vi "Read Col Data.vi"(7 "Section Name":string, 8 "error in (no error)":errorcluster, 10 "Col Header Name":string, 11 "Config Data":T1(array[cluster])) -> (0 "error out":errorcluster, 1 "Column Data":string[](array[string]), 3 "Config Data dup":T1(array[cluster]), 4 "Key Find?":bool)   [LabVIEW 2020, in "GUCalibration2.lvlib"]
uses:
  GUCalibration2.lvlib
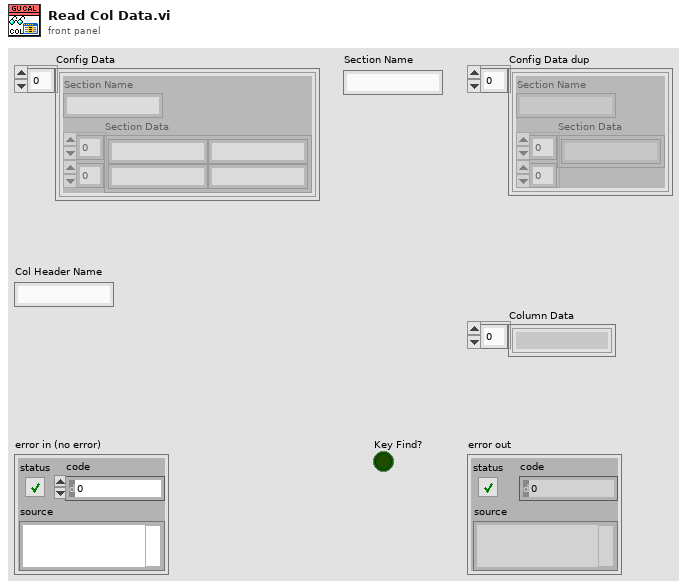
[diagram p1: front panel]
types:
  T1 = cluster{"Section Name":string, "Section Data":string[][]}[]
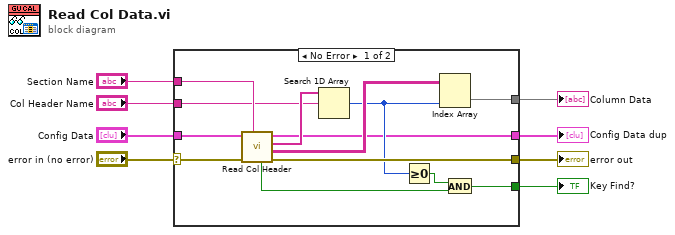
[diagram p0: block diagram]
diagram:
  n1 = case shown="No Error" "error in (no error)" {
    selector: "error in (no error)" -> [w19 w23]
    tunnel: "Section Name" -> [w20 _]
    tunnel: "Config Data" -> [w21 w22]
    tunnel: [w15 w23] -> w5
    tunnel: [w10 w22] -> w4
    tunnel: [w11 _] -> w3
    tunnel: [w9 _] -> w2
    tunnel: "Col Header Name" -> [w17 _]
    frame No Error {
      n2 = call "Read Col Header.vi"("Section Name"=w20, "error in (no error)"=w19, "Config Data"=w21) -> ("error out"=w15:errorcluster, "Data"=w16:string[][], "Column Header"=w18:string[], "Config Data dup"=w10:T1, "Section Find?"=w12:bool)  [unwired: 4 in]
      n3 = Search 1D Array(1D array=w18, element=w17) -> (index of element=w14:i32)  [unwired: 1 in]
      n4 = Greater Or Equal To 0?(x=w14) -> (x >= 0?=w13:bool)
      n5 = Index Array(array=w16, index (col)=w14) -> (element=w9:string[])  [unwired: 1 in]
      n6 = And(x=w13, y=w12) -> (x .and. y?=w11:bool)
    }
    frame Error {
    }
  }
  "error out" <- w5
  "Column Data" <- w2
  "Config Data dup" <- w4
  "Key Find?" <- w3
